vi "BK Precision 5491B Read Reference Measurement.vi"() -> ()   [LabVIEW 2020]
doc: "This example shows how to setup and enable reference and made a relative measurement."
uses:
  <instrlib>/BK Precision 5491B/BK Precision 5491B.lvlib
panel:
  out "Primary Measurement":dbl
  in  "Reference Value (0.00001)":dbl=1e-05 min=1e-05 max=20000000.0 format="%.5f"
  in  "Set Reference Method (0: Reference)":u16(ring) items=["Reference", "Input"]
  in  "Serial Configuration":T1={"Baud Rate"=9600, "Parity"=0, "Data Bits"=8, "Stop Bits"=10, "Flow Control"=0} {"Flow Control" items=["None", "XON/XOFF", "RTS/CTS", "XON/XOFF & RTS/CTS", "DTR/DSR", "XON/XOFF & DTR/DSR"]; "Stop Bits" items=["1.0"=10, "1.5"=15, "2.0"=20]; "Data Bits" items=["8"=8]; "Parity" items=["None", "Odd", "Even", "Mark", "Space"]; "Baud Rate" items=["300"=300, "600"=600, "1200"=1200, "2400"=2400, "4800"=4800, "9600"=9600, "19200"=19200]}
  in  "VISA resource name":refnum<visa-resource-name>
  # "(c) 2016 B&K Precision Corporation.  ALL RIGHTS RESERVED."
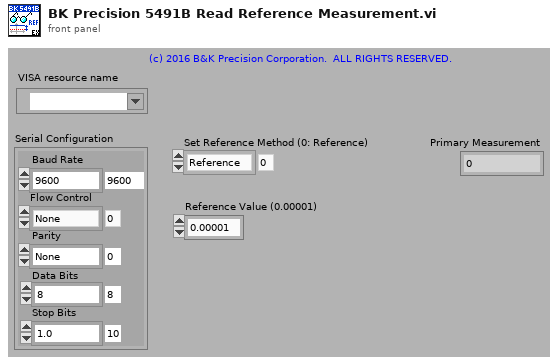
[diagram p1: front panel]
types:
  T1 = cluster{"Baud Rate":u32, "Parity":u16, "Data Bits":u16, "Stop Bits":u16, "Flow Control":u16}
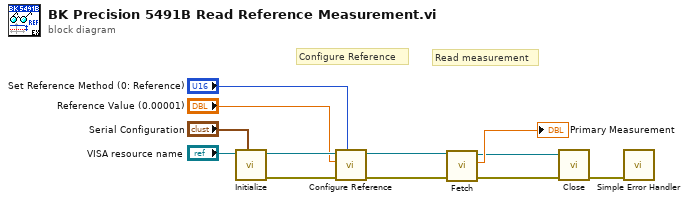
[diagram p0: block diagram]
diagram:
  # "Read measurement"
  # "Configure Reference"
  n1 = call <instrlib>:"Initialize.vi"("Serial Configuration"="Serial Configuration", "VISA resource name"="VISA resource name") -> ("error out"=w8:errorcluster, "VISA resource name out"=w9:refnum<visa-resource-name>)  [unwired: 8 in]
  n2 = call <instrlib>:"Configure Reference.vi"("Set Reference Method (0: Reference)"="Set Reference Method (0: Reference)", "error in (no error)"=w8, "Reference Value (0.00001)"="Reference Value (0.00001)", "VISA resource name"=w9) -> ("error out"=w4:errorcluster, "VISA resource name out"=w5:refnum<visa-resource-name>)  [unwired: 6 in]
  n3 = call <instrlib>:"Fetch.vi"("error in (no error)"=w4, "VISA resource name"=w5) -> ("error out"=w1:errorcluster, "Primary Measurement"=→"Primary Measurement":dbl, "VISA resource name out"=w2:refnum<visa-resource-name>)  [unwired: 6 in, 1 out]
  n4 = call <instrlib>:"Close.vi"("error in (no error)"=w1, "VISA resource name"=w2) -> ("error out"=w11:errorcluster)  [unwired: 9 in]
  n5 = call <vilib>:"Simple Error Handler.vi"("error in (no error)"=w11) -> ()  [unwired: 4 in, 5 out]
